vi "Get Board Id by handle.vi"(10 "board handle":u32, 11 "hw_data in":T1) -> (0 "port handles":u32[](array[numeric]), 1 "boardId":u32, 2 "key not found":bool, 3 "hw_data out":T1)   [LabVIEW 2020, in "AIM664LV.lvlib"]
uses:
  AIM664LV.lvlib
  _controls/hwEntry_data.ctl
  _controls/hwEntryBoardHandleMap.ctl
  _controls/hwEntryBoardResource.ctl
  _controls/hwEntryPortResource.ctl
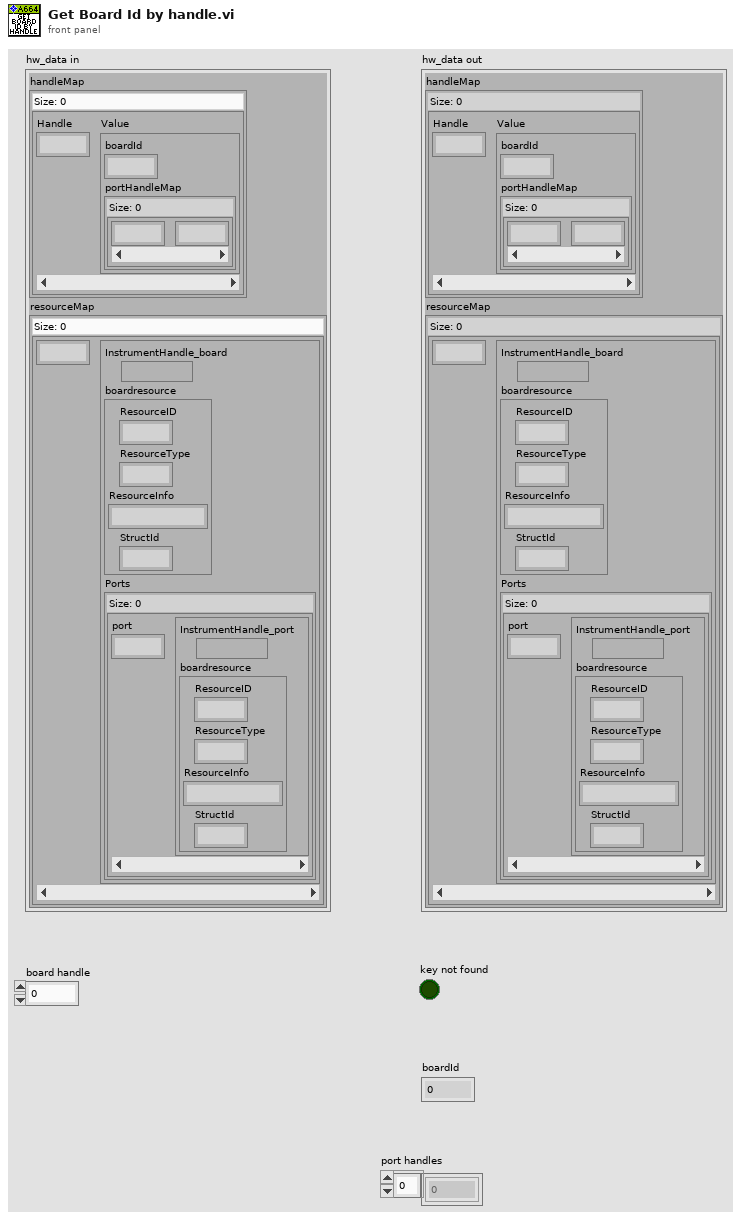
[diagram p1: front panel]
types:
  T1 = typedef "AIM664LV.lvlib/hwEntry_data.ctl" = cluster{"handleMap":map{u32, T2}, "resourceMap":map{u32, T3}}
  T2 = typedef "AIM664LV.lvlib/hwEntryBoardHandleMap.ctl" = cluster{"boardId":u32, "portHandleMap":map{u32, u32}}
  T3 = typedef "AIM664LV.lvlib/hwEntryBoardResource.ctl" = cluster{"InstrumentHandle_board":u32, "boardresource":cluster{"ResourceID":u32, "ResourceType":u32, "ResourceInfo":string, "StructId":u32}, "Ports":map{u32, T4}}
  T4 = typedef "AIM664LV.lvlib/hwEntryPortResource.ctl" = cluster{"InstrumentHandle_port":u32, "boardresource":cluster{"ResourceID":u32, "ResourceType":u32, "ResourceInfo":string, "StructId":u32}}
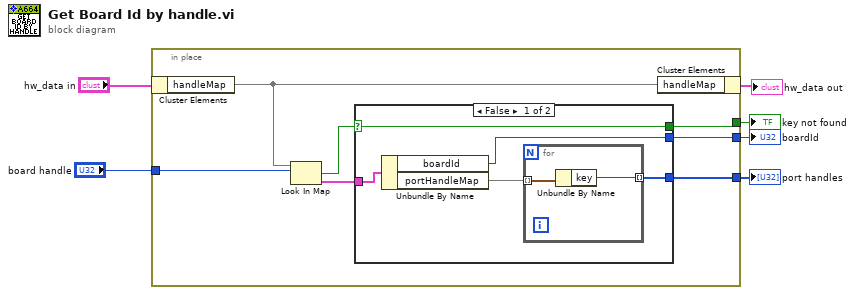
[diagram p0: block diagram]
diagram:
  n1 = in-place {
    in-place-border: "board handle" -> [w13]
    in-place-border: [w9] -> w3
    in-place-border: [w8] -> w2
    in-place-border: [w7] -> w1
    n2 = in-place-cluster #1("hw_data in") -> ("handleMap"=w10:map{u32, T2})
    n3 = Look In Map(map=w10, key=w13) -> (key not found?=w11:bool, value=w12:T2)  [unwired: 1 in]
    n4 = case shown="False" w11 {
      selector: w11 -> [w14 w21]
      tunnel: w12 -> [w18 _]
      tunnel: [w17 _] -> w9
      tunnel: [w15 _] -> w8
      tunnel: [w14 w21] -> w7
      frame False {
        n5 = Unbundle By Name(w18) -> ("boardId"=w17:u32, "portHandleMap"=w16:map{u32, u32})
        n6 = for {
          tunnel: w16 -> [w20] mode=indexing
          tunnel: [w19] -> w15 mode=indexing
          n7 = Unbundle By Name(w20) -> ("key"=w19:u32)
        }
      }
      frame True {
      }
    }
    n8 = in-place-cluster #1("handleMap"=w10) -> (→"hw_data out":T1)
  }
  "boardId" <- w3
  "port handles" <- w2
  "key not found" <- w1
